vi "ex10_signal processing.vi"() -> ()   [LabVIEW 2018]
uses:
  <vilib>/Analysis/3filter.llb/Filter Passband Type.ctl
  <vilib>/express/express analysis/Spectral/Block/exnSpectralBlock spectral measurements RMS poly.vi
  <vilib>/express/express analysis/Spectral/Block/exnSpectralBlock spectral measurements RMS WFM.vi
  <vilib>/Analysis/3filter.llb/Butterworth Filter (DBL).vi
  <vilib>/express/express analysis/Spectral/XNode/ExpressSpectralMeasurementsBlockNode.xnode
  <vilib>/Analysis/NI_AALBase.lvlib
panel:
  in  "high cutoff freq: fh":dbl=0.45000000000000007 format="%0.2f"
  out "Waveform Graph 2":dbl[](graph)
  in  "low cutoff freq: fl":dbl=0.12500000000000006 format="%0.4f"
  in  "filter type":T1
  in  "Noise amplitude":dbl=0.6
  out "Waveform Chart 3":dbl[](graph)
  in  "Frequency":dbl=100.0
  in  "stop 2":bool
  out "Waveform Chart 2":dynamicdata(graph)
  in  "frequency":dbl
  in  "amplitude":dbl
  in  "samples":i32
  out "Waveform Graph":cluster{"f0":dbl, "df":dbl, "magnitude":dbl[]}(graph)
  in  "stop":bool
  out "Waveform Chart":dbl[](graph)
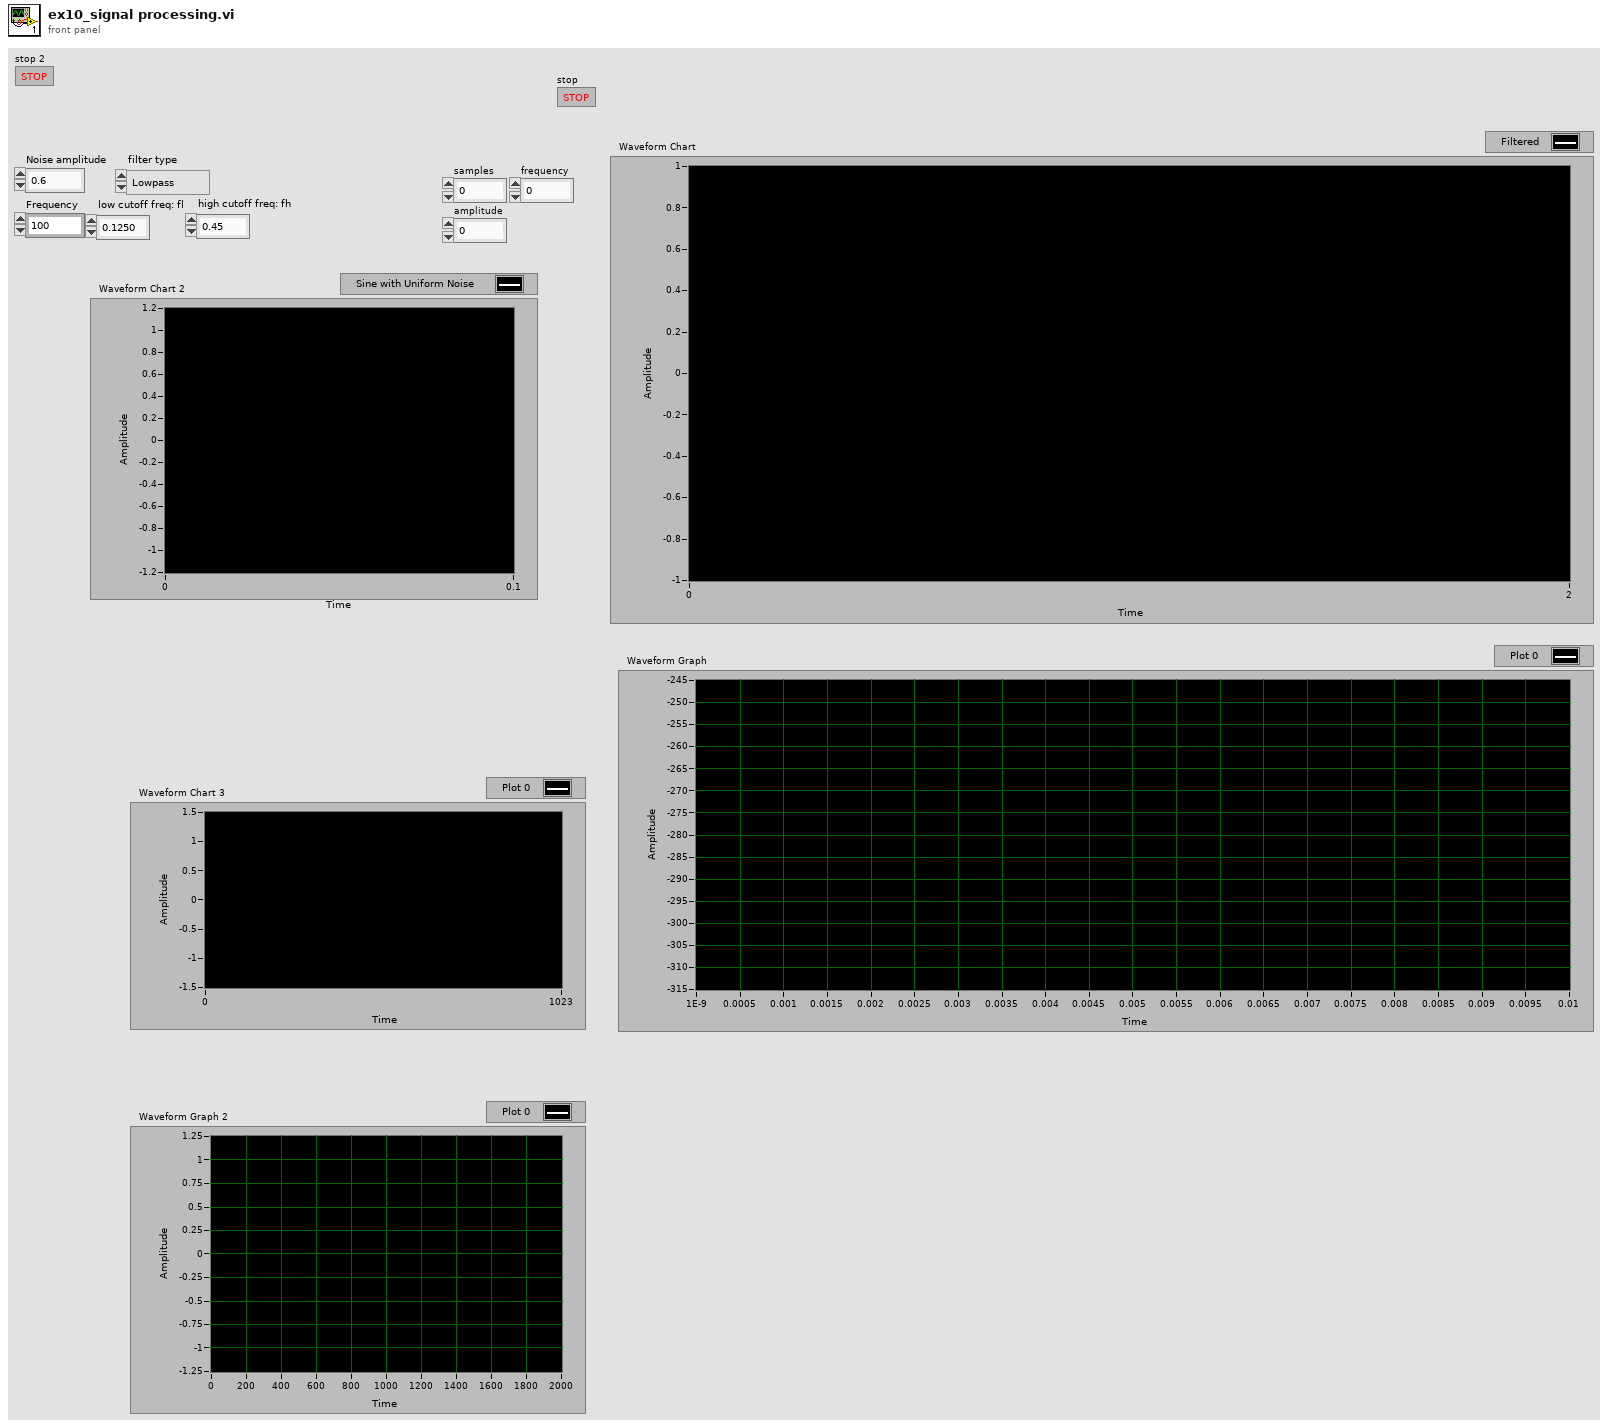
[diagram p1: front panel]
types:
  T1 = typedef "NI_AALBase.lvlib/Filter Passband Type.ctl" = enum32{"Lowpass", "Highpass", "Bandpass", "Bandstop"}
  T2 = cluster{"averaging mode":u16, "weighting mode":u16, "number of averages":u32}
  T3 = cluster{"dB On (F)":bool, "unwrap phase (F)":bool, "convert to degree (F)":bool}
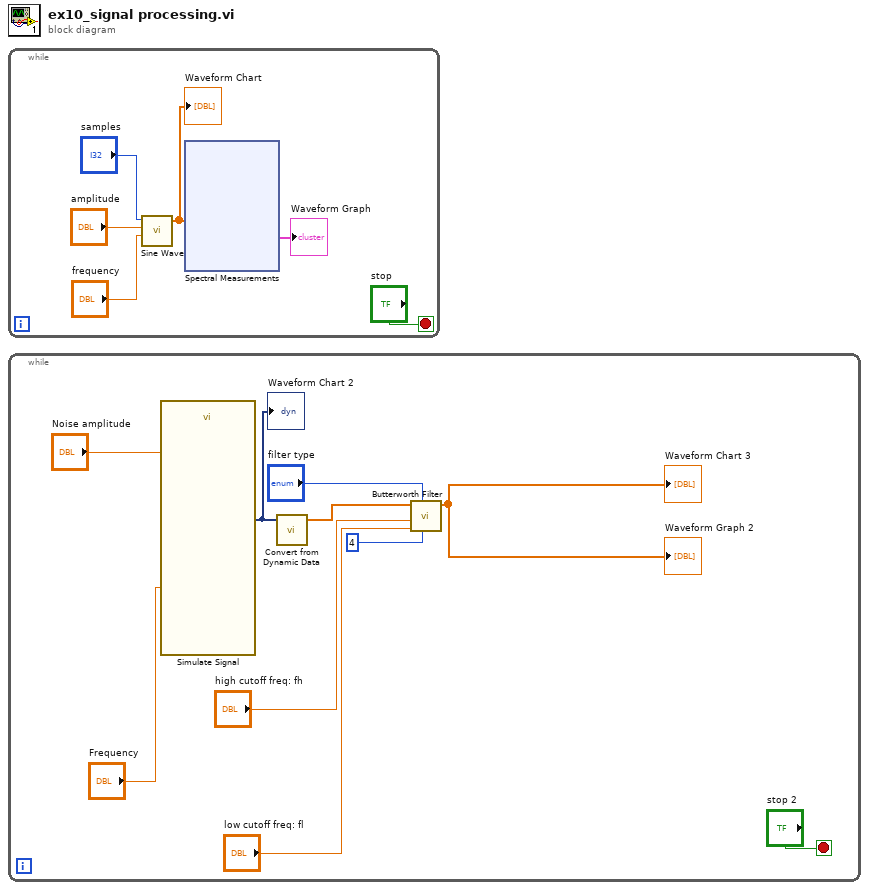
[diagram p0: block diagram]
diagram:
  n1 = while {
    stop <- "stop" stop-if-true
    n2 = call <vilib>:"Sine Wave.vi"("samples"="samples", "amplitude"="amplitude", "frequency"="frequency") -> ("sine wave"=w2:dbl[])  [unwired: 2 in, 2 out]
    "Waveform Chart" <- w2
    n3 = xnode "Spectral Measurements"("Signals"=w2) -> ("FFT - (RMS)"=→"Waveform Graph":cluster{"f0":dbl, "df":dbl, "magnitude":dbl[]})  [unwired: 1 in, 2 out]
  }
  n4 = while {
    stop <- "stop 2" stop-if-true
    n5 = call "Simulate Signal"("Frequency"="Frequency", "Noise amplitude"="Noise amplitude") -> ("Sine with Uniform Noise"=w24:dynamicdata)  [unwired: 12 in, 1 out]
    "Waveform Chart 2" <- w24
    n6 = call "Convert from Dynamic Data"("Dynamic Data Type"=w24) -> ("Array"=w23:dbl[])  [unwired: 3 in]
    n7 = call-poly <vilib>:"Butterworth Filter.vi"("order"=4, "filter type"="filter type", "low cutoff freq: fl"="low cutoff freq: fl", "high cutoff freq: fh"="high cutoff freq: fh", "X"=w23) -> ("Filtered X"=→"Waveform Chart 3" →"Waveform Graph 2":dbl[])  [unwired: 3 in, 1 out]
  }
